vi "Alazar_conTrig - ATS-SDK.vi"(3 "error in (no error)":errorcluster, 4 "Trigger":T1 {"Coupling" items=["DC 1 MOhm", "AC 1 MOhm", "DC 50 Ohm", "AC 50 Ohm"]; "Slope" items=["Positive", "Negative"]; "Level" format="%.2f"; "Source" items=["Chan 1", "External"]}, 5 "Voltage Scale":dbl(ring)=2.0 items=["8 V"=8.0, "4 V"=4.0, "2 V"=2.0, "800 mV"=0.8, "400 mV"=0.4, "200 mV"=0.2, "80 mV"=0.08], 6 "Handle in":u32) -> (0 "error out":errorcluster, 2 "Handle_Out":u32)   [LabVIEW 2022 SP3]
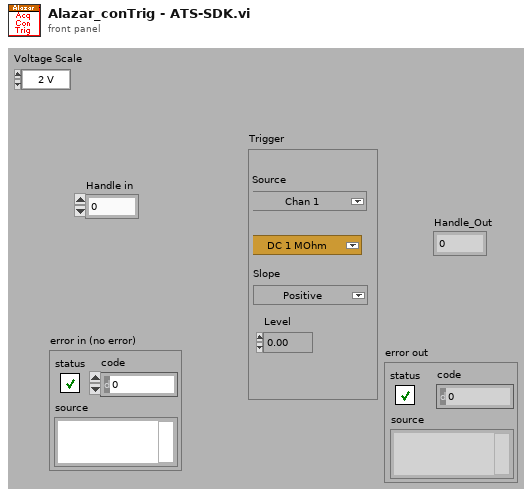
[diagram p1: front panel]
types:
  T1 = cluster{"Source":u16, "Coupling":u16, "Slope":u16, "Level":dbl}
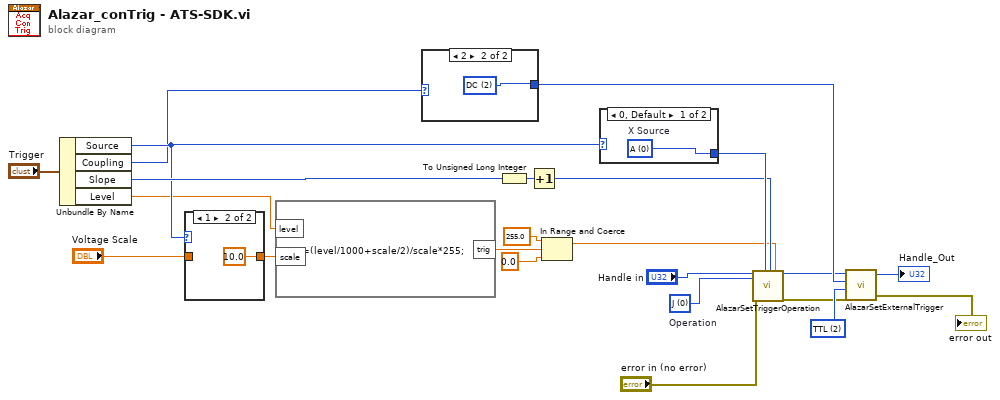
[diagram p0: block diagram]
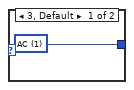
[diagram p2: hidden frame]
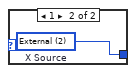
[diagram p4: hidden frame]
diagram:
  w4 = u32 0 items=["J", "K", "J OR K", "J AND K", "J XOR K", "J AND NOT K", "NOT J AND K"]  # Operation
  w11 = u32 2 items=["5 V", "1 V", "TTL"] ("Range")
  n1 = Unbundle By Name("Trigger") -> ("Source"=w18:u16, "Coupling"=w13:u16, "Slope"=w22:u16, "Level"=w17:dbl)
  n2 = case shown="1" w18 {
    tunnel: "Voltage Scale" -> [w24 _]
    tunnel: [w24 10.0 ("lower limit")] -> w16
    frame 0, Default {
    }
    frame 1 {
    }
  }
  n3 = formula code="trig=(level/1000+scale/2)/scale*255;"("level"=w17, "scale"=w16) -> ("trig"=w15:dbl)
  n4 = case shown="2" w13 {
    tunnel: [w26 w27] -> w10
    frame 3, Default {
      w26 = u32 1 items=["AC"=1, "DC"=2] ("Coupling")
    }
    frame 2 {
      w27 = u32 2 items=["AC"=1, "DC"=2] ("Coupling")
    }
  }
  n5 = To Unsigned Long Integer(number=w22) -> (unsigned 32bit integer=w21:u32)
  n6 = Increment(x=w21) -> (x+1=w6:u32)
  n7 = In Range and Coerce(upper limit=255.0, x=w15, lower limit=0.0) -> (coerced(x)=w5:dbl)  [unwired: 1 out]
  n8 = case shown="0, Default" w18 {
    tunnel: [w28 w29] -> w7
    frame 0, Default {
      w28 = u32 0 items=["A", "B", "External", "Disable", "C", "D"]  # X Source
    }
    frame 1 {
      w29 = u32 2 items=["A", "B", "External", "Disable", "C", "D"]  # X Source
    }
  }
  n9 = call "AlazarSetTriggerOperation.vi"("Handle"="Handle in", "Trigger Operation"=w4, "error in (no error)"="error in (no error)", "Source 1"=w7, "Slope 1"=w6, "Level 1"=w5) -> ("Handle"=w8:u64, "error out"=w3:errorcluster)  [unwired: 11 in, 1 out]
  n10 = call "AlazarSetExternalTrigger.vi"("error in (no error)"=w3, "Range ID"=w11, "Coupling ID"=w10, "Handle"=w8) -> ("error out"=→"error out":errorcluster, "Handle"=→"Handle_Out":u64)  [unwired: 1 out]
